vi "aoc-2025-d05-2.vi"() -> ()   [LabVIEW 2020]
panel:
  out "size of final ranges":i32
  out "iterations":i32
  out "size of input ranges":i32
  out "input ranges":cluster{"[0]":u64, "[1]":u64}[](array[cluster])
  out "final ranges":cluster{"[0]":u64, "[1]":u64}[](array[cluster])
  out "ans":u64
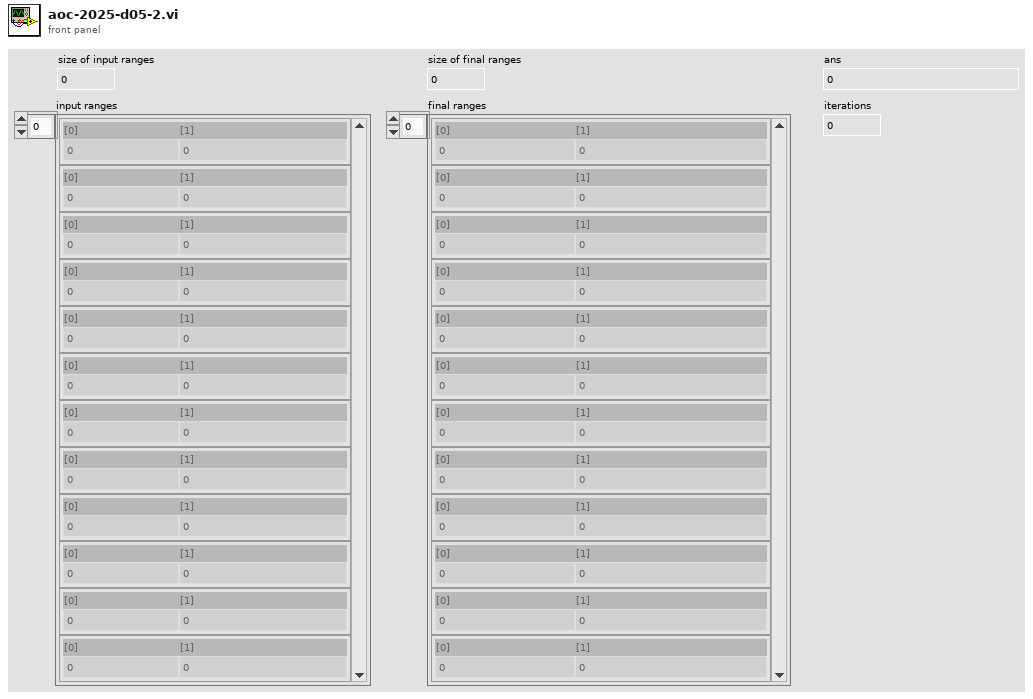
[diagram p1: front panel]
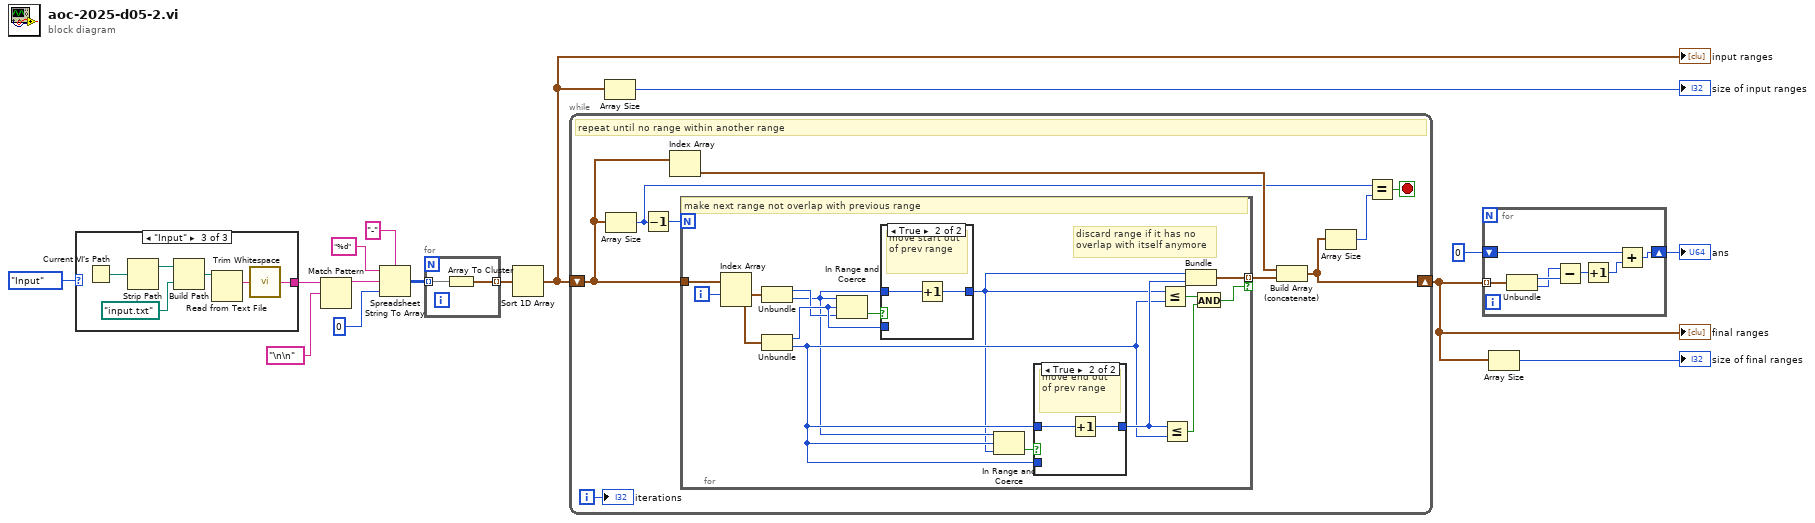
[diagram p0: block diagram]
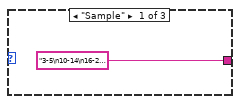
[diagram p4: hidden frame]
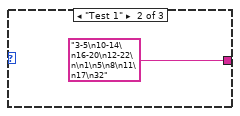
[diagram p5: hidden frame]
diagram:
  n1 = case shown="\"Input\"" enum16{"Sample", "Input", "Test 1"}."Input" {
    tunnel: ["3-5\n10-14\n16-20\n12-18\n\n1\n5\n8\n11\n17\n32" "3-5\n10-14\n16-20\n12-22\n\n1\n5\n8\n11\n17\n32" w18] -> w8
    frame "Sample" {
    }
    frame "Test 1" {
    }
    frame "Input" {
      n2 = Current VI's Path() -> (path=w23:path)
      n3 = Strip Path(path=w23) -> (stripped path=w22:path)  [unwired: 1 out]
      n4 = Build Path(base path=w22, name or relative path=path "input.txt") -> (appended path=w20:path)
      n5 = Read from Text File(file (use dialog)=w20) -> (text=w19:string)  [unwired: 3 in, 3 out]
      n6 = call <vilib>:"Trim Whitespace.vi"("string"=w19) -> ("trimmed string"=w18:string)  [unwired: 1 in]
    }
  }
  n7 = Match Pattern(string=w8, regular expression="\n\n") -> (before substring=w14:string)  [unwired: 1 in, 3 out]
  n8 = Spreadsheet String To Array(delimiter (Tab)="-", format string="%d", spreadsheet string=w14, array type (2D Dbl)=u64 0) -> (array=w10:u64[][])
  n9 = for {
    tunnel: w10 -> [w25] mode=indexing
    tunnel: [w24] -> w4 mode=indexing
    n10 = Array To Cluster(array=w25) -> (cluster=w24:cluster{"[0]":u64, "[1]":u64})
  }
  n11 = Sort 1D Array(array=w4) -> (sorted array=w3:cluster{"[0]":u64, "[1]":u64}[])
  "input ranges" <- w3
  n12 = while {
    shift-right: [w30] -> w2
    shift-left: w3 -> [w33]
    i -> [w26]
    stop <- w31 stop-if-true
    # "repeat until no range within another range"
    n13 = Array Size(array=w33) -> (size(s)=w27:i32)
    n14 = Decrement(x=w27) -> (x-1=w34:i32)
    n15 = Index Array(array=w33) -> (element=w29:cluster{"[0]":u64, "[1]":u64})  [unwired: 1 in]
    n16 = for {
      N: w34 -> [_]
      tunnel: w33 -> [w50]
      tunnel: [w43] -> w32 mode=indexing if=w40
      i -> [w49]
      # "discard range if it has no \noverlap with itself anymore"
      # "make next range not overlap with previous range"
      n17 = Index Array(array=w50, index #1=w49) -> (element #1=w48:cluster{"[0]":u64, "[1]":u64}, element #2=w47:cluster{"[0]":u64, "[1]":u64})  [unwired: 1 in]
      n18 = Unbundle(w48) -> ("[0]"=w37:u64, "[1]"=w36:u64)
      n19 = Unbundle(w47) -> ("[0]"=w39:u64, "[1]"=w38:u64)
      n20 = In Range and Coerce(upper limit=w36, x=w39, lower limit=w37) -> (In Range?=w46:bool)  [unwired: 1 out]
      n21 = case shown="True" w46 {
        tunnel: w36 -> [_ w56]
        tunnel: [w54 w55] -> w35
        tunnel: w39 -> [w54 _]
        frame False {
        }
        frame True {
          # "move start out of prev range"
          n22 = Increment(x=w56) -> (x+1=w55:u64)
        }
      }
      n23 = In Range and Coerce(upper limit=w36, x=w38, lower limit=w35) -> (In Range?=w45:bool)  [unwired: 1 out]
      n24 = case shown="True" w45 {
        tunnel: w38 -> [_ w53]
        tunnel: [w51 w52] -> w44
        tunnel: w38 -> [w51 _]
        frame False {
        }
        frame True {
          # "move end out of prev range"
          n25 = Increment(x=w53) -> (x+1=w52:u64)
        }
      }
      n26 = Less Or Equal?(x=w35, y=w38) -> (x <= y?=w42:bool)
      n27 = Less Or Equal?(x=w44, y=w38) -> (x <= y?=w41:bool)
      n28 = Bundle("[0]"=w35, "[1]"=w44) -> (w43:cluster{"[0]":u64, "[1]":u64})  [unwired: 1 in]
      n29 = And(x=w42, y=w41) -> (x .and. y?=w40:bool)
    }
    n30 = Build Array (concatenate)(w29, w32) -> (w30:cluster{"[0]":u64, "[1]":u64}[])
    n31 = Array Size(array=w30) -> (size(s)=w28:i32)
    n32 = Equal?(x=w27, y=w28) -> (x = y?=w31:bool)
    "iterations" <- w26
  }
  "final ranges" <- w2
  n33 = Array Size(array=w3) -> (size(s)=→"size of input ranges":i32)
  n34 = for {
    tunnel: w2 -> [w60] mode=indexing
    shift-right: [w57] -> w9
    shift-left: u64 0 -> [w59]
    n35 = Unbundle(w60) -> ("[0]"=w62:u64, "[1]"=w61:u64)
    n36 = Subtract(x=w61, y=w62) -> (x-y=w63:u64)
    n37 = Increment(x=w63) -> (x+1=w58:u64)
    n38 = Add(x=w59, y=w58) -> (x+y=w57:u64)
  }
  "ans" <- w9
  n39 = Array Size(array=w2) -> (size(s)=→"size of final ranges":i32)
